vi "sub Menu save file.vi"(8 "error in (no error)":errorcluster, 11 "LF2R IDE in":refnum<class "LF2R IDE.lvclass">) -> (0 "error out":errorcluster, 3 "LF2R IDE out":refnum<class "LF2R IDE.lvclass">)   [LabVIEW 2018, in "LF2R IDE.lvlib" / "LF2R IDE.lvclass"]
uses:
  LF2R IDE.lvclass
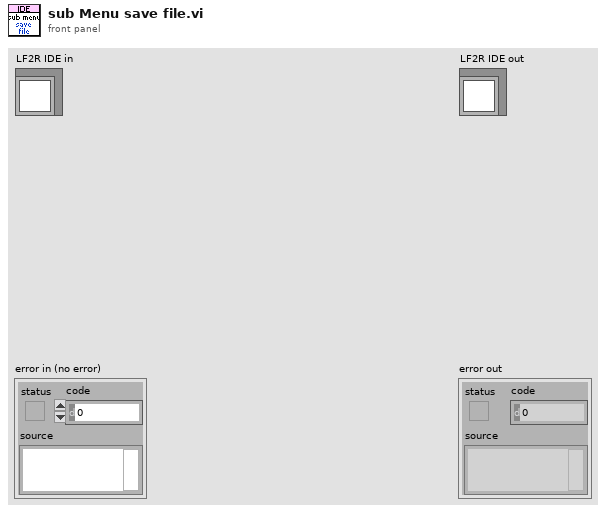
[diagram p1: front panel]
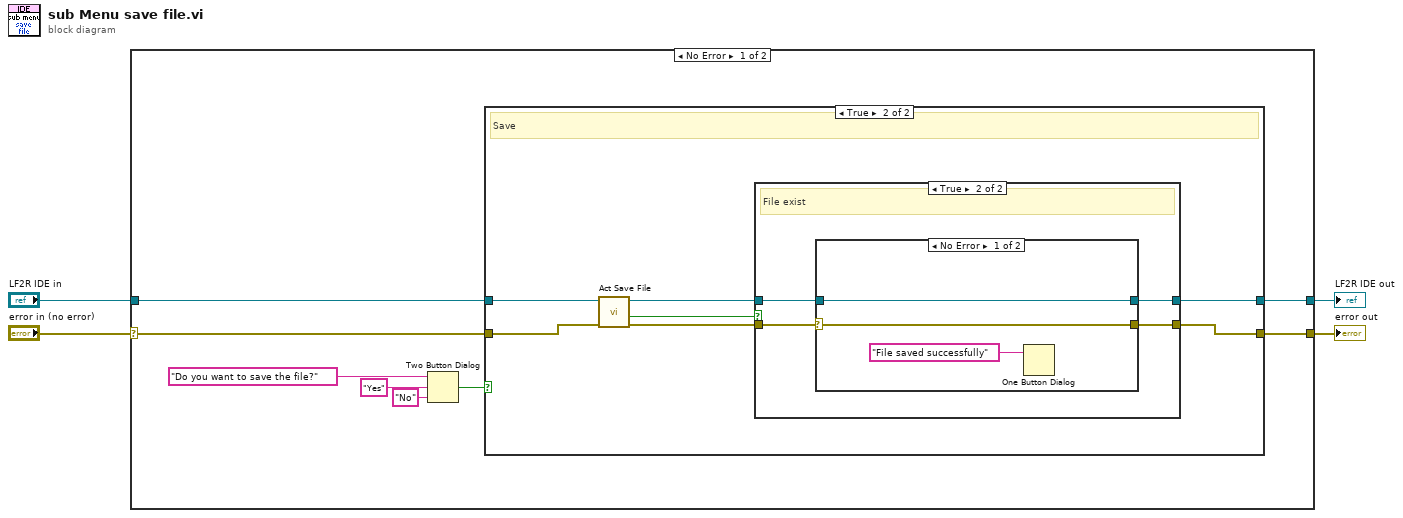
[diagram p0: block diagram]
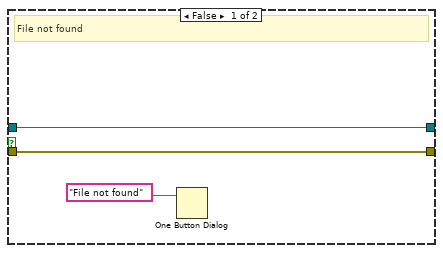
[diagram p3: hidden frame]
diagram:
  n1 = case shown="No Error" "error in (no error)" {
    selector: "error in (no error)" -> [w5 w35]
    tunnel: [w12 w35] -> w3
    tunnel: [w10 w34] -> w1
    tunnel: "LF2R IDE in" -> [w11 w34]
    frame No Error {
      n2 = Two Button Dialog(message="Do you want to save the file?", 1:"No" ("F button name (\"Cancel\")"), 2:"Yes" ("T button name (\"OK\")")) -> (T button?=w6:bool)
      n3 = case shown="True" w6 {
        tunnel: [w13 w15] -> w12
        tunnel: w11 -> [w14 w21]
        tunnel: [w14 w16] -> w10
        tunnel: w5 -> [w13 w20]
        frame False {
        }
        frame True {
          # "Save"
          n4 = call "Act Save File.vi"("error in (no error)"=w20, "LF2R IDE in"=w21) -> ("error out"=w17:errorcluster, "File Exist?"=w19:bool, "LF2R IDE out"=w18:refnum<class "LF2R IDE.lvclass">)  [unwired: 7 in]
          n5 = case shown="True" w19 {
            tunnel: w18 -> [w23 w26]
            tunnel: w17 -> [w22 w28]
            tunnel: [w22 w27] -> w15
            tunnel: [w23 w25] -> w16
            frame False {
              # "File not found"
              n6 = One Button Dialog(message="File not found") -> ()  [unwired: 1 in, 1 out]
            }
            frame True {
              # "File exist"
              n7 = case shown="No Error" w28 {
                selector: w28 -> [w30 w32]
                tunnel: [w30 w32] -> w27
                tunnel: w26 -> [w29 w33]
                tunnel: [w29 w33] -> w25
                frame No Error {
                  n8 = One Button Dialog(message="File saved successfully") -> ()  [unwired: 1 in, 1 out]
                }
                frame Error {
                }
              }
            }
          }
        }
      }
    }
    frame Error {
    }
  }
  "error out" <- w3
  "LF2R IDE out" <- w1
